vi "forexample.vi"() -> ()   [LabVIEW 2017]
panel:
  in  "stop":bool
  out "Contador double":dbl
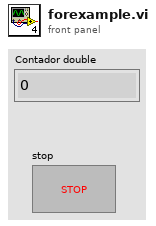
[diagram p1: front panel]
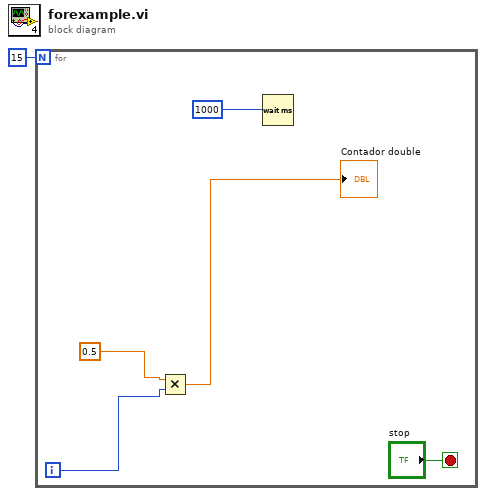
[diagram p0: block diagram]
diagram:
  n1 = for {
    N: 15 -> [_]
    i -> [w5]
    stop <- "stop" stop-if-true
    n2 = Multiply(x=0.5, y=w5) -> (x*y=→"Contador double":dbl)
    n3 = Wait (ms)(milliseconds to wait=1000) -> ()  [unwired: 1 out]
  }
